vi "SV Cells automatico.vi"(4 "error in":errorcluster, 5 "Offset Row":u16(knob)=3 min=1 scale=1.0..30.0, 6 "Offset Column":u16(knob)=2 min=1 scale=1.0..30.0, 7 "Refnum Cluster In":T1) -> (0 "error out":errorcluster, 1 "Final cells":cluster{"Column":i32, "Row":i32}, 2 "Datos":string[][](array[string]), 3 "Refnum Cluster Out":T1)   [LabVIEW 2010]
doc: "Se extraen automaticamente las celdas del archivo deseado sin necesidad de conocer cuantos datos hay, se es posible poner un offset que permita dar un colchon en caso de que no todas las celdas en la hoja esten cubiertas."
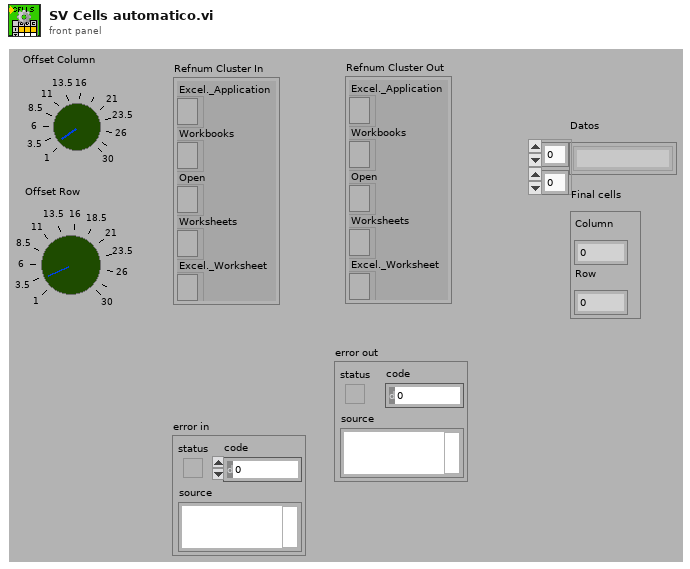
[diagram p1: front panel]
types:
  T1 = cluster{"Excel._Application":refnum<k7>, "Workbooks":refnum<k7>, "Open":refnum<k7>, "Worksheets":refnum<k7>, "Excel._Worksheet":refnum<k7>}
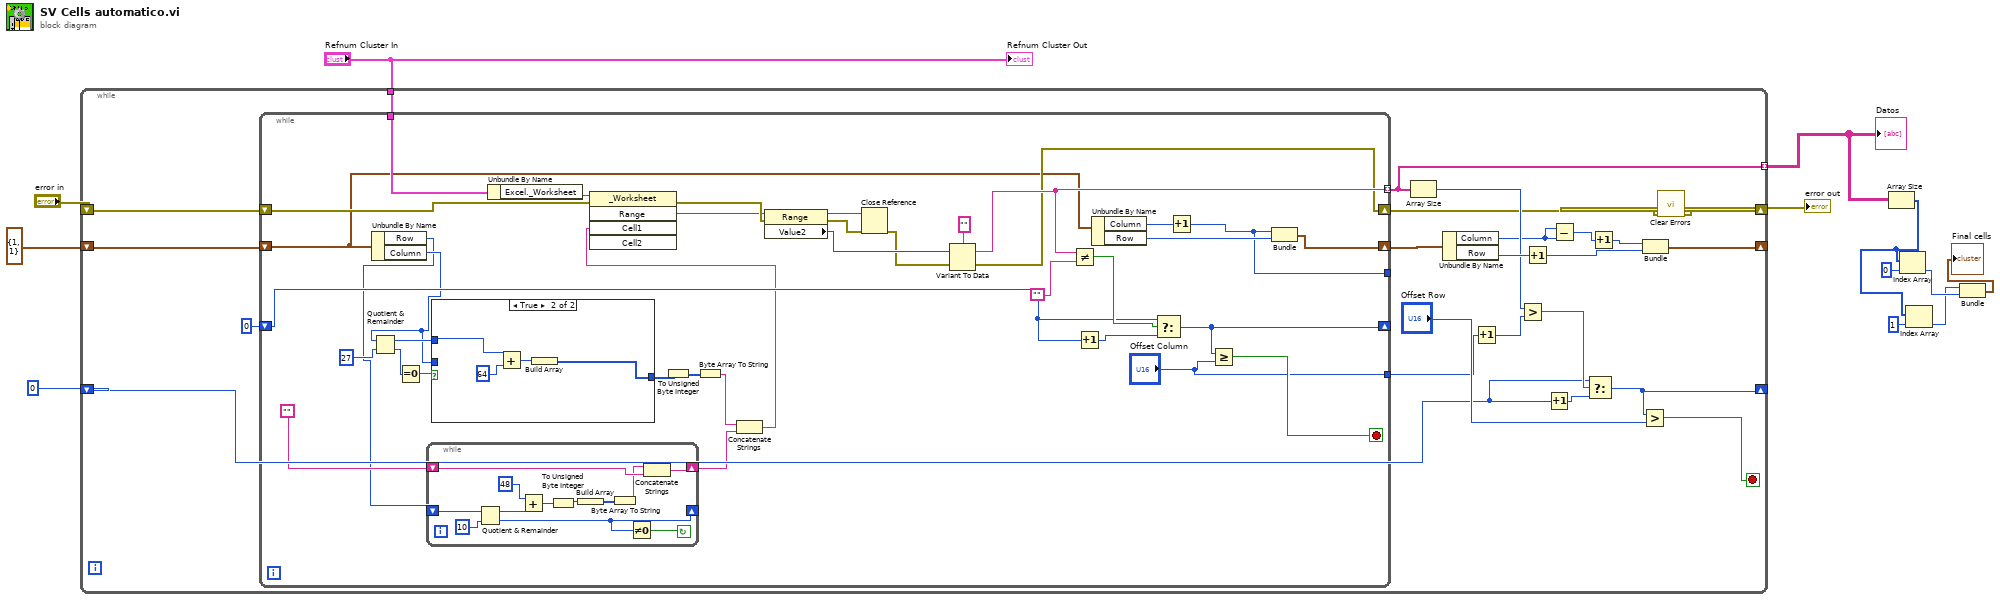
[diagram p0: block diagram]
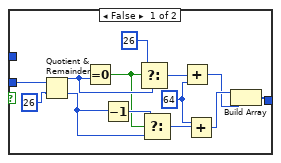
[diagram p2: hidden frame]
diagram:
  n1 = while {
    tunnel: "Refnum Cluster In" -> [w34]
    shift-right: [w25] -> _
    shift-left: cluster{"Column":i32, "Row":i32} {"Column"=1, "Row"=1} ("Start") -> [w33]
    shift-right: [w18] -> w10
    shift-left: "error in" -> [w35]
    shift-right: [w29] -> _
    shift-left: u16 0 -> [w15]
    tunnel: [w24] -> w7 mode=indexing
    stop <- w30 stop-if-true
    n2 = while {
      tunnel: w34 -> [w62]
      shift-right: [w60] -> w28
      shift-left: w33 -> [w52]
      tunnel: [w59] -> w24 mode=indexing
      shift-right: [w56] -> _
      shift-left: u16 0 -> [w54]
      shift-right: [w53] -> w17
      shift-left: w35 -> [w71]
      tunnel: [w49] -> _
      tunnel: ["Offset Column"] -> w13
      stop <- w57 stop-if-true
      n3 = Unbundle By Name(w52) -> ("Row"=w37:i32, "Column"=w38:i32)
      n4 = Quotient & Remainder(x=w38, y=27) -> (x-y*floor(x/y)=w44:i32, floor(x/y)=w45:i32)
      n5 = Equal To 0?(x=w45) -> (x = 0?=w46:bool)
      n6 = while {
        shift-left: w37 -> [w83]
        shift-right: [w74] -> _
        shift-left: "" -> [w73]
        shift-right: [w76] -> w39
        stop <- w75 continue-if-true
        n7 = Quotient & Remainder(x=w83, y=10) -> (x-y*floor(x/y)=w81:i32, floor(x/y)=w74:i32)
        n8 = Add(x=48, y=w81) -> (x+y=w79:i32)
        n9 = To Unsigned Byte Integer(number=w79) -> (unsigned 8bit integer=w78:u8)
        n10 = Build Array(w78) -> (w77:u8[])
        n11 = Byte Array To String(unsigned byte array=w77) -> (string=w72:string)
        n12 = Not Equal To 0?(x=w74) -> (x != 0?=w75:bool)
        n13 = Concatenate Strings(w72, w73) -> (w76:string)
      }
      n14 = case shown="True" w46 {
        tunnel: w38 -> [w96 _]
        tunnel: w44 -> [_ w100]
        tunnel: [w85 w99] -> w43
        frame False {
          w84 = 64
          n15 = Quotient & Remainder(x=w96, y=26) -> (x-y*floor(x/y)=w93:i32, floor(x/y)=w90:i32)
          n16 = Equal To 0?(x=w93) -> (x = 0?=w91:bool)
          n17 = Decrement(x=w90) -> (x-1=w92:i32)
          n18 = Select(t=26, s=w91, f=w93) -> (s? t:f=w89:i32)
          n19 = Select(t=w92, s=w91, f=w90) -> (s? t:f=w88:i32)
          n20 = Add(x=w89, y=w84) -> (x+y=w86:i32)
          n21 = Add(x=w84, y=w88) -> (x+y=w87:i32)
          n22 = Build Array(w87, w86) -> (w85:i32[])
        }
        frame True {
          n23 = Add(x=w100, y=64) -> (x+y=w97:i32)
          n24 = Build Array(w97) -> (w99:i32[])
        }
      }
      n25 = Unbundle By Name(w62) -> ("Excel._Worksheet"=w63:refnum<k7>)
      n26 = To Unsigned Byte Integer(number=w43) -> (unsigned 8bit integer=w42:u8[])
      n27 = Byte Array To String(unsigned byte array=w42) -> (string=w40:string)
      n28 = Concatenate Strings(w40, w39) -> (w36:string)
      n29 = invoke class="_Worksheet" method="Range"(reference=w63, error in=w71, "Cell1"=w36) -> (error out=w70:errorcluster, "Range"=w69:refnum<k7>)  [unwired: 2 in, 3 out]
      n30 = property class="Range"(reference=w69, error in=w70) -> (reference out=w68:refnum<k7>, error out=w67:errorcluster, "Value2"=w66:variant)
      n31 = Close Reference(reference=w68, error in (no error)=w67) -> (error out=w65:errorcluster)
      n32 = Variant To Data(error in=w65, Variant=w66, type="") -> (error out=w53:errorcluster, data=w59:string)
      n33 = Not Equal?(x=w59, y="") -> (x != y?=w58:bool)
      n34 = Increment(x=w54) -> (x+1=w55:u16)
      n35 = Unbundle By Name(w52) -> ("Column"=w51:i32, "Row"=w50:i32)
      n36 = Select(t=w54, s=w58, f=w55) -> (s? t:f=w56:u16)
      n37 = Increment(x=w51) -> (x+1=w49:i32)
      n38 = Greater Or Equal?(x=w56, y="Offset Column") -> (x >= y?=w57:bool)
      n39 = Bundle(w49, "Row"=w50) -> (w60:cluster{i32, "Row":i32})  [unwired: 1 in]
    }
    n40 = Array Size(array=w24) -> (size(s)=w23:i32)
    n41 = Unbundle By Name(w28) -> ("Column"=w21:i32, "Row"=w27:i32)
    n42 = Increment(x=w13) -> (x+1=w14:u16)
    n43 = Greater?(x=w23, y=w14) -> (0:w22:bool)
    n44 = Increment(x=w27) -> (x+1=w26:i32)
    n45 = Increment(x=w15) -> (x+1=w31:u16)
    n46 = Subtract(x=w21, y=w21) -> (x-y=w19:i32)
    n47 = Select(t=w15, s=w22, f=w31) -> (s? t:f=w29:u16)
    n48 = Increment(x=w19) -> (x+1=w20:i32)
    n49 = Greater?(x=w29, y="Offset Row") -> (0:w30:bool)
    n50 = Bundle(w20, w26) -> (w25:cluster{i32, i32})  [unwired: 1 in]
    n51 = call <vilib>:"Clear Errors.vi"("error in (no error)"=w17) -> ("error out"=w18:errorcluster)  [unwired: 6 in]
  }
  "error out" <- w10
  "Datos" <- w7
  n52 = Array Size(array=w7) -> (size(s)=w4:i32[])
  n53 = Index Array(array=w4, index=0) -> (element=w2:i32)
  n54 = Index Array(array=w4, index=1) -> (element=w1:i32)
  n55 = Bundle(w1, w2) -> (→"Final cells":cluster{i32, i32})  [unwired: 1 in]
  "Refnum Cluster Out" <- "Refnum Cluster In"
